vi "SCAN TIME.vi"(1 "Time in":string) -> (0 "Time out":string)   [LabVIEW 2020]
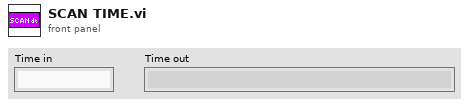
[diagram p1: front panel]
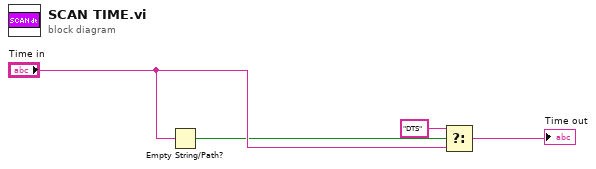
[diagram p0: block diagram]
diagram:
  n1 = Empty String/Path?(string/path="Time in") -> (empty?=w1:bool)
  n2 = Select(t="DTS", s=w1, f="Time in") -> (s? t:f=→"Time out":string)
